vi "Object Tracking.vi"() -> ()   [LabVIEW 2018]
doc: "Object Tracking: This example is an object tracking example that can recognize and track specific objects or targets in a continuous image sequence."
uses:
  vi.lib/VIRobotics/opencv_yiku/ctls/ColorConversionCodes.ctl
  vi.lib/VIRobotics/opencv_yiku/ctls/color.ctl
  vi.lib/VIRobotics/opencv_yiku/Mat/Mat_8U/Mat_8U.lvclass
  D:/Program Files/company/National Instruments/LabVIEW 2018/vi.lib/addons/VIRobotics/opencv_yiku/Mat/Mat/Mat.lvclass
  vi.lib/VIRobotics/opencv_yiku/Mat/Create_Mat_8U.vi
  vi.lib/VIRobotics/opencv_yiku/Cap/Cap.lvclass
  vi.lib/VIRobotics/opencv_yiku/opencv_yiku.lvlib
  vi.lib/VIRobotics/opencv_yiku/Mat/Mat/Mat.lvclass
panel:
  out "img":picture
  out "res":picture
  out "edge":picture
  out "mask":picture
  in  "stop":bool
  # "Overview:  Demonstrates how to convert a BGR image to HSV, we can use this to extract a colored object.In our example, we will try to extract a blue colored object.\nRequirements: Windows.\nInstructions: \n1.Make sure your compuuter has a camera.\n2. Run the VI"
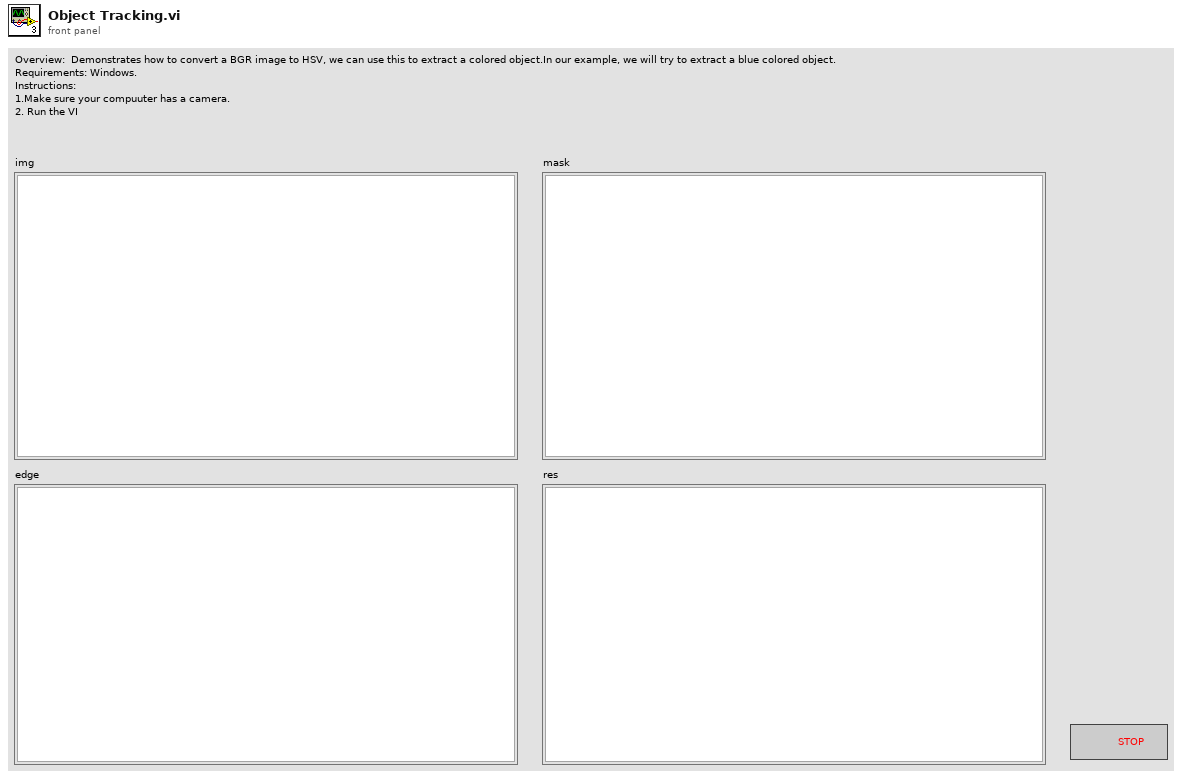
[diagram p1: front panel]
types:
  T1 = typedef "opencv_yiku.lvlib/ColorConversionCodes.ctl" = enum32{"COLOR_BGR2BGRA", "COLOR_BGRA2BGR", "COLOR_BGR2RGBA", "COLOR_RGBA2BGR", "COLOR_BGR2RGB", "COLOR_BGRA2RGBA", "COLOR_BGR2GRAY", "COLOR_RGB2GRAY", "COLOR_GRAY2BGR", "COLOR_GRAY2BGRA", "COLOR_BGRA2GRAY", "COLOR_RGBA2GRAY", "COLOR_BGR2BGR565", "COLOR_RGB2BGR565", "COLOR_BGR5652BGR", "COLOR_BGR5652RGB", "COLOR_BGRA2BGR565", "COLOR_RGBA2BGR565", "COLOR_BGR5652BGRA", "COLOR_BGR5652RGBA", "COLOR_GRAY2BGR565", "COLOR_BGR5652GRAY", "COLOR_BGR2BGR555", "COLOR_RGB2BGR555", "COLOR_BGR5552BGR", "COLOR_BGR5552RGB", "COLOR_BGRA2BGR555", "COLOR_RGBA2BGR555", "COLOR_BGR5552BGRA", "COLOR_BGR5552RGBA", "COLOR_GRAY2BGR555", "COLOR_BGR5552GRAY", "COLOR_BGR2XYZ", "COLOR_RGB2XYZ", "COLOR_XYZ2BGR", "COLOR_XYZ2RGB", "COLOR_BGR2YCrCb", "COLOR_RGB2YCrCb", "COLOR_YCrCb2BGR", "COLOR_YCrCb2RGB", "COLOR_BGR2HSV", "COLOR_RGB2HSV", "42", "43", "COLOR_BGR2Lab", "COLOR_RGB2Lab"}
  T2 = typedef "opencv_yiku.lvlib/color.ctl" = cluster{"c1":u8, "c2":u8, "c3":u8}
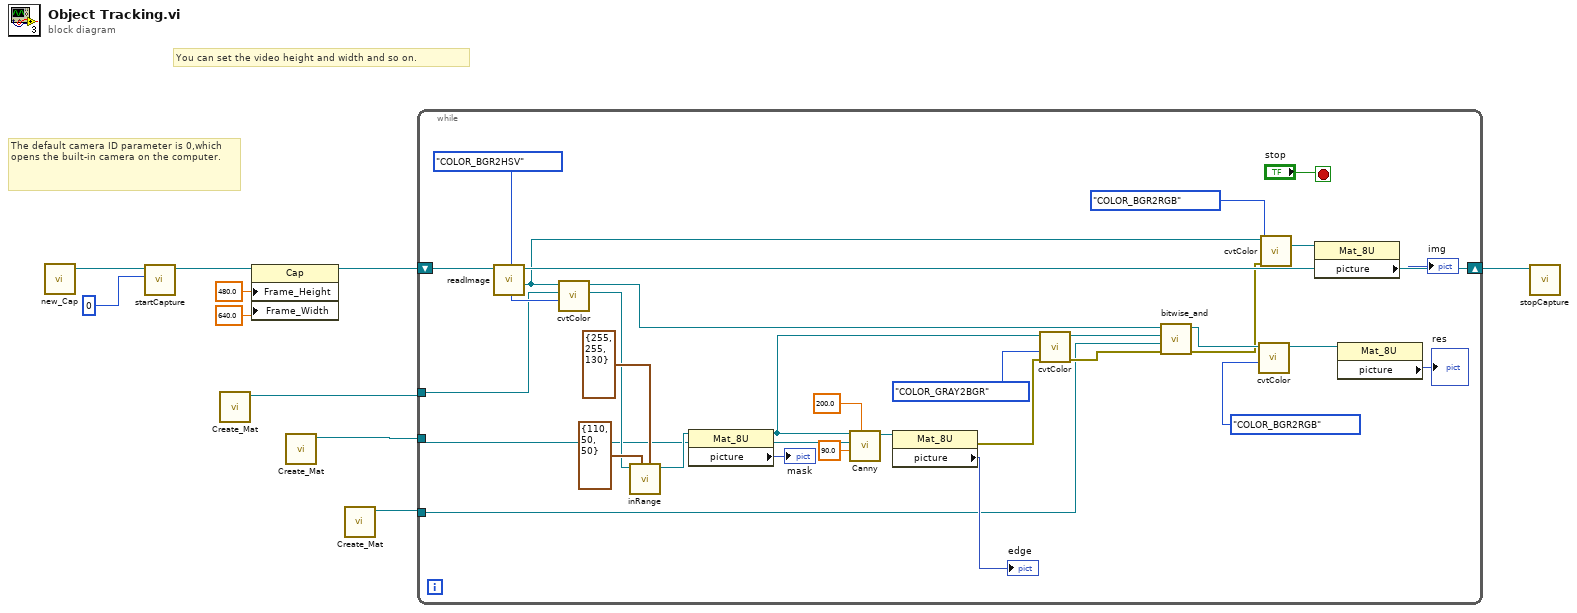
[diagram p0: block diagram]
diagram:
  # "You can set the video height and width and so on."
  # "The default camera ID parameter is 0,which opens the built-in camera on the computer."
  n1 = call "new_Cap.vi"() -> ("Cap out"=w10:refnum<class "Cap.lvclass">)  [unwired: 10 in, 1 out]
  n2 = call "startCapture.vi"("cameraID"=0, "Cap in"=w10) -> ("Cap out"=w7:refnum<class "Cap.lvclass">)  [unwired: 8 in, 1 out]
  n3 = call-poly "Create_Mat.vi"() -> ("Mat_8U_out"=w3:refnum<class "Mat_8U.lvclass">)  [unwired: 10 in, 1 out]
  n4 = property class="Cap"(reference=w7, "Frame_Height"=480.0, "Frame_Width"=640.0) -> (reference out=w6:refnum<class "Cap.lvclass">)  [unwired: 1 in, 1 out]
  n5 = call-poly "Create_Mat.vi"() -> ("Mat_8U_out"=w2:refnum<class "Mat_8U.lvclass">)  [unwired: 10 in, 1 out]
  n6 = call-poly "Create_Mat.vi"() -> ("Mat_8U_out"=w1:refnum<class "Mat_8U.lvclass">)  [unwired: 10 in, 1 out]
  n7 = while {
    shift-right: [w40] -> w8
    shift-left: w6 -> [w41]
    tunnel: w3 -> [w15]
    tunnel: w2 -> [w14]
    tunnel: w1 -> [w13]
    stop <- "stop" stop-if-true
    n8 = call "readImage.vi"("Cap in"=w41) -> ("Mat out"=w11:refnum<class "Mat_8U.lvclass">, "Cap out"=w40:refnum<class "Cap.lvclass">)  [unwired: 8 in, 1 out]
    n9 = call "cvtColor.vi"("dstCn"=ColorConversionCodes."COLOR_BGR2HSV", "dst"=w15, "src"=w11) -> ("dst out"=w16:refnum<class "Mat_8U.lvclass">, "src out"=w12:refnum<class "Mat_8U.lvclass">)  [unwired: 6 in, 1 out]
    n10 = call "inRange.vi"("higherb"=T2 {"c1"=255, "c2"=255, "c3"=130}, "lowerb"=T2 {"c1"=110, "c2"=50, "c3"=50}, "Mat"=w16) -> ("Mat_out"=w17:refnum<class "Mat_8U.lvclass">)  [unwired: 6 in, 2 out]
    n11 = property class="Mat_8U"(reference=w17) -> (reference out=w29:refnum<class "Mat_8U.lvclass">, "picture"=→"mask":picture)  [unwired: 1 in, 1 out]
    n12 = call "Canny.vi"("threshold2"=200.0, "threshold1"=90.0, "dst in"=w14, "Mat in"=w29) -> ("dst out"=w32:refnum<class "Mat_8U.lvclass">)  [unwired: 6 in, 1 out]
    n13 = property class="Mat_8U"(reference=w32) -> (error out=w28:errorcluster, "picture"=→"edge":picture)  [unwired: 1 in, 1 out]
    n14 = call "cvtColor.vi"("error in (no error)"=w28, "dstCn"=ColorConversionCodes."COLOR_GRAY2BGR", "src"=w29) -> ("error out"=w27:errorcluster, "src out"=w25:refnum<class "Mat_8U.lvclass">)  [unwired: 6 in, 1 out]
    n15 = call "bitwise_and.vi"("error in (no error)"=w27, "dst"=w13, "src2"=w25, "src1"=w12) -> ("error out"=w18:errorcluster, "dst out"=w19:refnum<class "Mat_8U.lvclass">)  [unwired: 6 in]
    n16 = call "cvtColor.vi"("dstCn"=ColorConversionCodes."COLOR_BGR2RGB", "src"=w19) -> ("src out"=w24:refnum<class "Mat_8U.lvclass">)  [unwired: 7 in, 2 out]
    n17 = call "cvtColor.vi"("error in (no error)"=w18, "dstCn"=ColorConversionCodes."COLOR_BGR2RGB", "src"=w11) -> ("dst out"=w20:refnum<class "Mat_8U.lvclass">)  [unwired: 6 in, 2 out]
    n18 = property class="Mat_8U"(reference=w20) -> ("picture"=→"img":picture)  [unwired: 1 in, 2 out]
    n19 = property class="Mat_8U"(reference=w24) -> ("picture"=→"res":picture)  [unwired: 1 in, 2 out]
  }
  n20 = call "stopCapture.vi"("Cap in"=w8) -> ()  [unwired: 10 in, 1 out]
